vi "Close.vi"(8 "error in (no error)":errorcluster, 10 "Data":variant) -> (0 "error out":errorcluster)   [LabVIEW 2014, in "Control Module.lvlib"]
uses:
  Control Module.lvlib
  Message.ctl
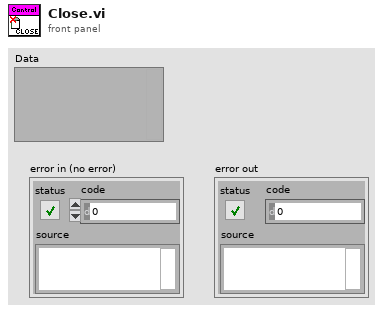
[diagram p1: front panel]
types:
  T1 = typedef "Control Module.lvlib/Message.ctl" = cluster{"Message":enum16{"Initialise", "Error", "Close"}, "Data":variant}
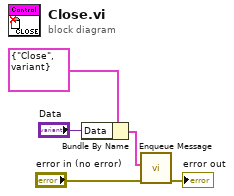
[diagram p0: block diagram]
diagram:
  n1 = Bundle By Name(cluster=T1 {"Message"=enum."Close", "Data"=variant} ("output cluster"), "Data"="Data") -> (w3:T1)
  n2 = call "Enqueue Message.vi"("error in (no error)"="error in (no error)", "output cluster"=w3) -> ("error out"=→"error out":errorcluster)  [unwired: 8 in, 1 out]
